vi "GEvt-Generate Interrupt Log.vi"(0 "CSM Global Log Event":T4, 1 "Current State":string, 2 "Arguments":string, 6 "Name (\"\" to Use UUID)":string, 10 "CSM:LogFilter.lvclass":refnum<class "LogFilter.lvclass">) -> (14 "CSM Global Log Event Out":T4, 16 "Event Data":T1={"Name (\"\" to Use UUID)"="", "Current State"="", "Arguments"="", "Source Message"={"‘State"="", "’Arguments"="", "’Error"={"status"=FALSE, "code"=0, "source"=""}}, "Source Module"="", "Complete(T)/Start(F)"=FALSE, "LogType"=enum."State Change", "Time Stamp"=timestamp(0 s since 1904-01-01)})   [LabVIEW 2017, in "Communicable State Machine.lvlib"]
doc: "### GEvt-Generate Interrupt Log.vi\n\n-- <b>Controls</b> --\n- <b>CSM Global Log Event</b>:\n- <b>Current State</b>:\n- <b>Arguments</b>:\n- <b>Name(\"\" to use uuid)</b>:\n- <b>CSM:LogFilter.lvclass</b>:\n\n-- <b>Indicators</b> --\n- <b>CSM Global Log Event out</b>:\n- <b>event data</b>:"
uses:
  Communicable State Machine.lvlib
  GEvt-Refs.ctl
  Typedef/_CSM_GlobalLog_MSG.ctl
  Typedef/_CSM_Response Source Message.ctl
  Typedef/_CSM_GlobalLog_MSG_TYPE.ctl
  LogFilter/LogFilter.lvclass
  LogFilter/LogFilter - Check.vi
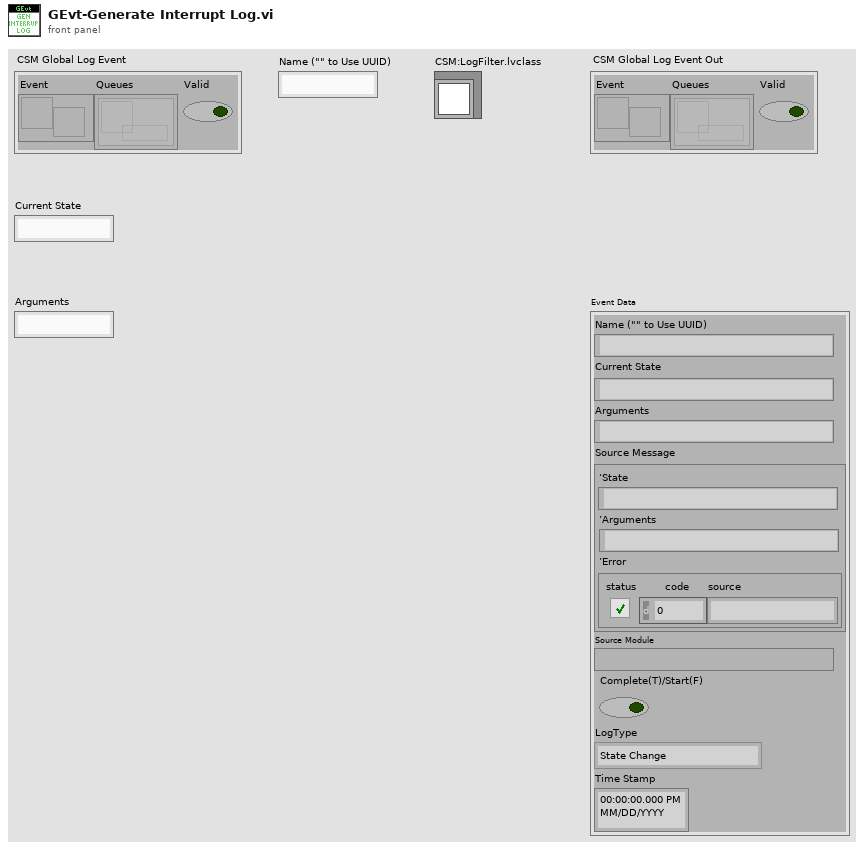
[diagram p1: front panel]
types:
  T1 = typedef "Communicable State Machine.lvlib/_CSM_GlobalLog_MSG.ctl" = cluster{"Name (\"\" to Use UUID)":string, "Current State":string, "Arguments":string, "Source Message":T2, "Source Module":string, "Complete(T)/Start(F)":bool, "LogType":T3, "Time Stamp":timestamp}
  T2 = typedef "Communicable State Machine.lvlib/_CSM_Response Source Message.ctl" = cluster{"‘State":string, "’Arguments":string, "’Error":errorcluster}
  T3 = typedef "Communicable State Machine.lvlib/_CSM_GlobalLog_MSG_TYPE.ctl" = enum16{"User Log", "State Change", "Status", "Interrupt", "Register", "Unregister", "Error Log", "Module Created", "Module Destroyed", "Async Message", "No-Rep Async Message", "Sync Message", "AsyncMsg Complete", "SyncMsg Complete"}
  T4 = typedef "Communicable State Machine.lvlib/GEvt-Refs.ctl" = cluster{"Event":refnum<user-event>, "Queues":refnum<queue>[], "Valid":bool}
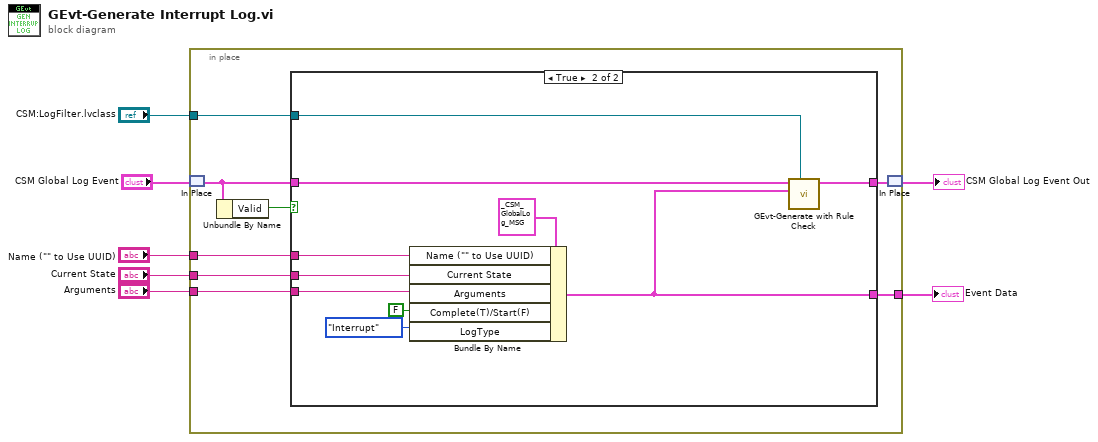
[diagram p0: block diagram]
diagram:
  n1 = in-place {
    in-place-border: [w14] -> w5
    in-place-border: "Name (\"\" to Use UUID)" -> [w13]
    in-place-border: "Current State" -> [w12]
    in-place-border: "Arguments" -> [w11]
    in-place-border: "CSM:LogFilter.lvclass" -> [w10]
    n2 = in-place-match #1("CSM Global Log Event") -> (w9:T4)
    n3 = Unbundle By Name(w9) -> ("Valid"=w8:bool)
    n4 = case shown="True" w8 {
      tunnel: w9 -> [w16 w26]
      tunnel: [w16 w25] -> w15
      tunnel: [_ w17] -> w14
      tunnel: w13 -> [_ w21]
      tunnel: w12 -> [_ w20]
      tunnel: w11 -> [_ w19]
      tunnel: w10 -> [_ w18]
      frame False {
      }
      frame True {
        n5 = Bundle By Name(cluster=T1 {"Name (\"\" to Use UUID)"="", "Current State"="", "Arguments"="", "Source Message"={"‘State"="", "’Arguments"="", "’Error"={"status"=FALSE, "code"=0, "source"=""}}, "Source Module"="", "Complete(T)/Start(F)"=FALSE, "LogType"=enum."State Change", "Time Stamp"=timestamp(0 s since 1904-01-01)} ("event data"), "Name (\"\" to Use UUID)"=w21, "Current State"=w20, "Arguments"=w19, "Complete(T)/Start(F)"=FALSE, "LogType"=_CSM_GlobalLog_MSG_TYPE."Interrupt" ("Type")) -> (w17:T1)
        n6 = call "GEvt-Generate with Rule Check.vi"("LogFilter In"=w18, "Event Data"=w17, "CSM Global Log Event In"=w26) -> ("CSM Global Log Event Out"=w25:T4)  [unwired: 8 in]
      }
    }
    n7 = in-place-match #1(w15) -> (→"CSM Global Log Event Out":T4)
  }
  "Event Data" <- w5
